vi "CANFD Get Bus Error.vi"(8 "error in (no error)":errorcluster, 9 "pCanBusError":cluster{"TEC":u8, "REC":u8, "Flags":u8}, 10 "CANIndex":u8, 11 "DevHandle":i32) -> (0 "error out":errorcluster, 1 "pCanBusError out":cluster{"TEC":u8, "REC":u8, "Flags":u8}, 3 "function return":i32)   [LabVIEW 2010, in "usb2canfd.lvlib"]
doc: "int WINAPI CANFD_GetBusError(int DevHandle, unsigned char CANIndex, CANFD_BUS_ERROR *pCanBusError);"
uses:
  usb2canfd.lvlib
  USB2XXX/trunk/USB2XXX/USB2XXX/vs2010/Release/USB2XXX.dll
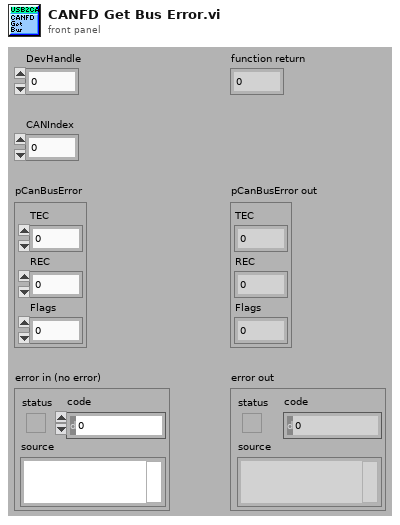
[diagram p1: front panel]
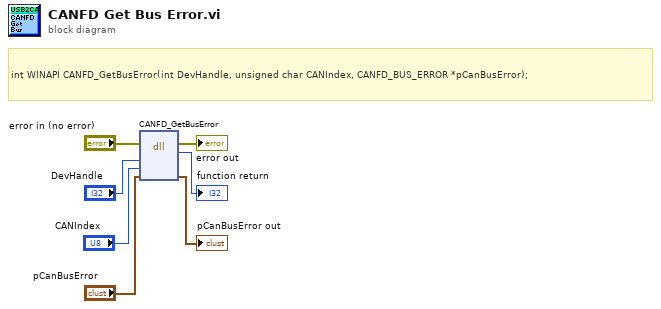
[diagram p0: block diagram]
diagram:
  # "int WINAPI CANFD_GetBusError(int DevHandle, unsigned char CANIndex, CANFD_BUS_ERROR *pCanBusError);"
  n1 = dll-call lib="E:/OtherWork/STM32/USB2XXX/trunk/USB2XXX/USB2XXX/vs2010/Release/USB2XXX.*" fn="CANFD_GetBusError"(error in="error in (no error)", "DevHandle"="DevHandle", "CANIndex"="CANIndex", "pCanBusError"="pCanBusError") -> (error out=→"error out":errorcluster, →"function return":i32, "pCanBusError"=→"pCanBusError out":cluster{"TEC":u8, "REC":u8, "Flags":u8})  [unwired: 4 in, 1 out]
